vi "Auto.vi"() -> ()   [LabVIEW 2013]
panel:
  in  "Auto Intake":dbl=2.318
  in  "Auto Arm":dbl=5.0
  in  "Auto Winch":dbl=0.616
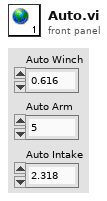
[diagram p1: front panel]
diagram:
